vi "Dequeue CTRL Element.vi"(8 "error in (no error)":errorcluster, 11 "CTRL Data Queue in":refnum<queue>) -> (0 "error out":errorcluster, 2 "Control Data":T1, 3 "CTRL Data Queue out":refnum<queue>)   [LabVIEW 2014, in "WINFAS 2 Data Queue.lvlib"]
uses:
  WINFAS 2 Data Queue.lvlib
  Control Data Cluster.ctl
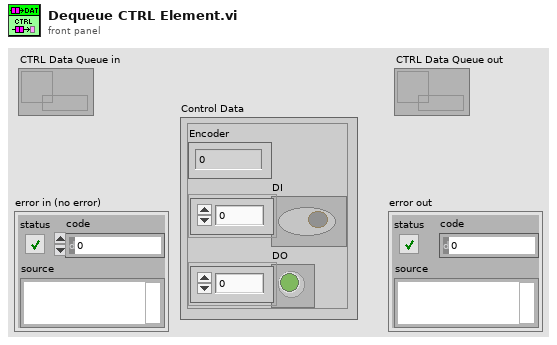
[diagram p1: front panel]
types:
  T1 = typedef "WINFAS 2 Data Queue.lvlib/Control Data Cluster.ctl" = cluster{"Encoder":sgl, "DI":bool[], "DO":bool[]}
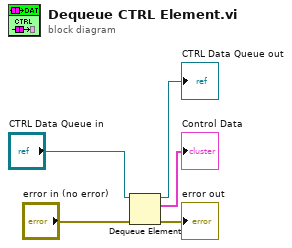
[diagram p0: block diagram]
diagram:
  n1 = Dequeue Element(queue="CTRL Data Queue in", error in (no error)="error in (no error)") -> (queue out=→"CTRL Data Queue out":refnum<queue>, element=→"Control Data":T1, error out=→"error out":errorcluster)  [unwired: 1 in, 1 out]
